vi "getValidPacketRange.vi"(11 "MQTTVersion in":refnum<class "MQTTVersion.lvclass">) -> (1 "Lower Range":u8=1 format="%02x", 2 "Upper Range":u8=14 format="%02x", 3 "MQTTVersion out":refnum<class "MQTTVersion.lvclass">)   [LabVIEW 2013, in "MQTT_Control_Packets.lvlib" / "MQTTVersion.lvclass"]
uses:
  MQTTVersion.lvclass
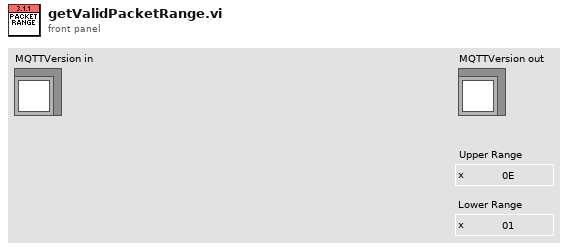
[diagram p1: front panel]
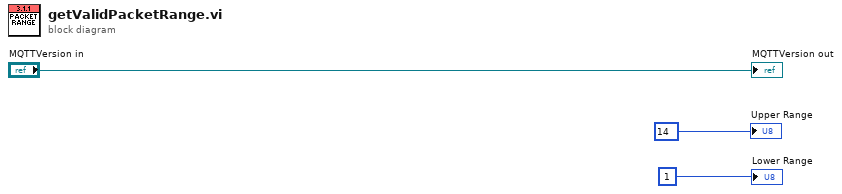
[diagram p0: block diagram]
diagram:
  "MQTTVersion out" <- "MQTTVersion in"
  "Upper Range" <- u8 14 ("Byte")
  "Lower Range" <- u8 1 ("Byte")
